vi "Speaker Array Calibration.vi"(11 "folder":path=path "D:/Data/Calibrations/SAL") -> ()   [LabVIEW 2020]
uses:
  SAC Config/SAC Config.xctl
  HRTF VIs/Typedefs/HRTF-Result.ctl
  Typedefs/SAC-Parameters.ctl
  HRTF VIs/Typedefs/HRTF-Waveform.ctl
  HRTF VIs/Typedefs/HRTF-Window.ctl
  HRTF VIs/Typedefs/HRTF-Window Type.ctl
  Typedefs/SAC-State.ctl
  Typedefs/SAC-Options.ctl
  Typedefs/SAC-Hardware Config (TDT).ctl
  PXI DAQ VIs/TDT VIs/Typedefs/TDT-Output source.ctl
  PXI DAQ VIs/TDT VIs/Typedefs/TDT-Device ID.ctl
  PXI DAQ VIs/TDT VIs/Typedefs/TDT-Device Config.ctl
  PXI DAQ VIs/TDT VIs/Typedefs/TDT-Input source.ctl
  HRTF VIs/Typedefs/HRTF-State Machine Action.ctl
  Typedefs/SAC-Runtime Data.ctl
  <vilib>/Analysis/2dsp.llb/Real FFT.vi
  <vilib>/Utility/miscctls.llb/LVBoundsTypeDef.ctl
  <vilib>/Analysis/NI_AALPro.lvlib
panel:
  in  "Measure":bool
  in  "Sensitivity (dB V/SPL)":dbl=128.0
  in  "Mic gain":dbl=128.0
  in  "Compute":bool
  in  "Window":T1={"Window"=0, "Length (ms)"=50.0, "Center (ms)"=50.0} {"Window" items=["None", "Rectangle", "Hanning"]}
  out "Result":T2
  out "StimDur":dbl format="%#_3g ms"
  in  "wftab":enum32{"Page 1", "Page 2"}(tab)
  in  "Freq Step (Hz)":dbl=50.0
  in  "Seed":i32=50
  in  "Order":i32=50
  in  "Attenuation (dB)":dbl=30.0
  in  "Sample Rate (Hz)":dbl=100000.0
  in  "Waveform":enum16{"Chirp", "MLS"}(ring)
  out "Progress":u8(slide) scale=0.0..2.0
  in  "Start":bool
  in  "Stop":bool
  in  "Config":i32(xcontrol)
  in  "Averages":i32=128
  in  "Data Tab":enum32{"Stimulus", "Response", "Calibrations"}(tab)
  out "StimPhase":cluster{i32, "dx":dbl, "Y":dbl[]}(graph)
  out "StimMag":cluster{i32, "dx":dbl, "Y":dbl[]}(graph)
  out "StimAutocorr":cluster{dbl, "dx":dbl, "Y":dbl[]}(graph) caption="Autocorrelation"
  out "Stimulus (time)":cluster{i32, "dx":dbl, "Y":dbl[]}(graph) caption="Amplitude"
  out "RespTime":cluster{"offset":dbl, "dx":dbl, "Y":dbl[]}(graph) caption="Amplitude"
  in  "RespFiles":u16(ring) items=["", "Speaker-az0", "Speaker-az90"]
  out "RespCorr":cluster{"offset":dbl, "dx":dbl, "Y":dbl[]}(graph) caption="Impulse Response"
  out "RespMag":cluster{"offset":dbl, "dx":dbl, "Y":dbl[]}(graph)
  out "RespPhase":cluster{"offset":dbl, "dx":dbl, "Y":dbl[]}(graph)
  out "Status":string
  in  "ASTFFiles":u16(ring) items=["", "Speaker-az-90", "Speaker-az0", "Speaker-az45", "Speaker-az90"]
  out "ASTFMag":cluster{"offset":dbl, "dx":dbl, "Y":dbl[]}(graph)
  out "ASTFPhase":cluster{"offset":dbl, "dx":dbl, "Y":dbl[]}(graph)
  out "ASIR":cluster{"offset":dbl, "dx":dbl, "Y":dbl[]}(graph) caption="Impulse Response"
  # "Speaker Array Calibration"
  # "Stimulus"
  # "ASTF"
  # "Response"
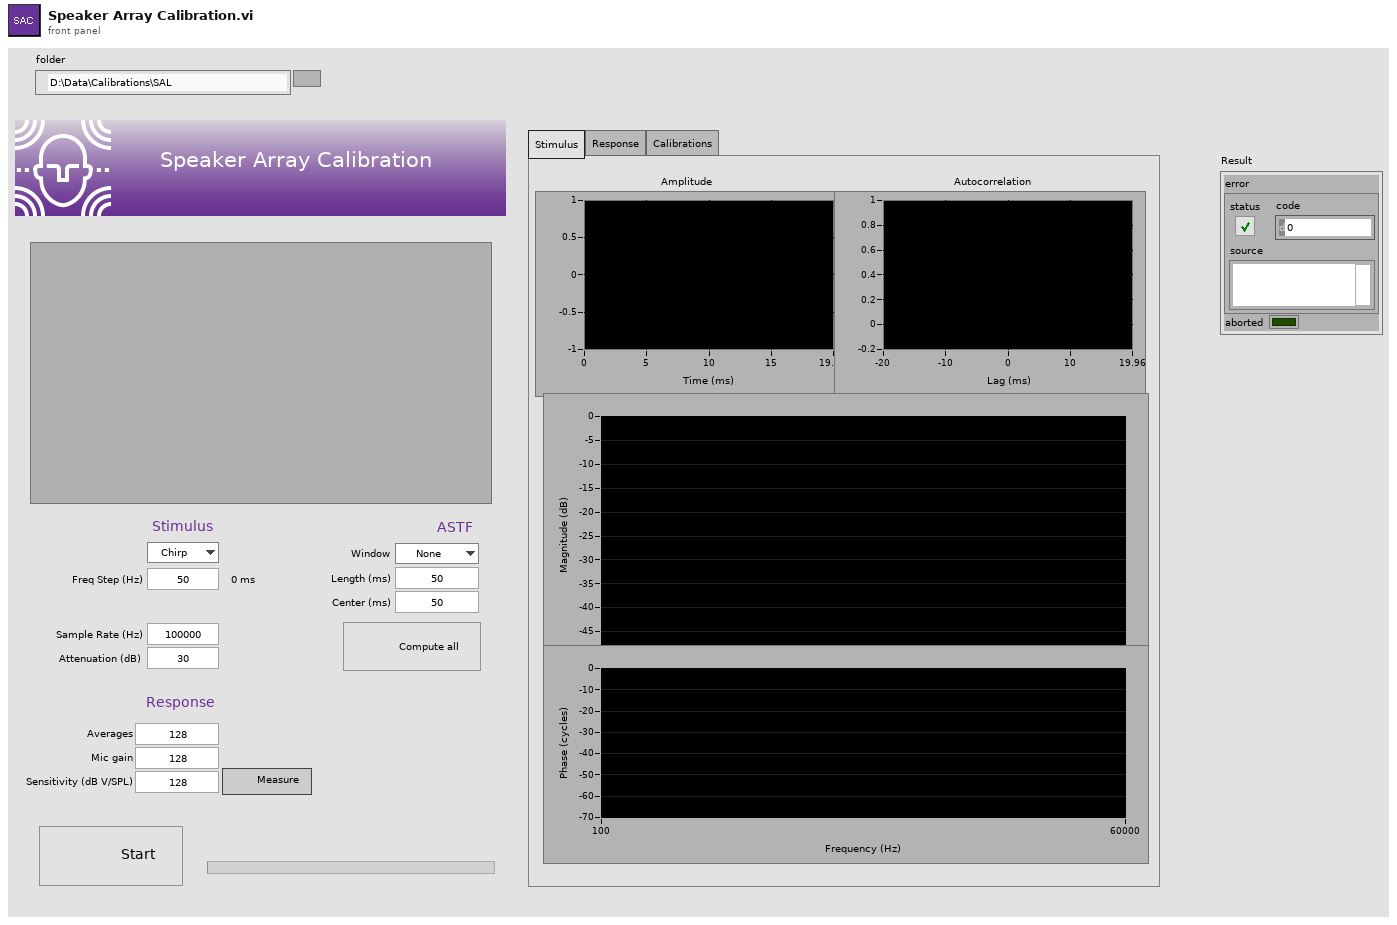
[diagram p1: front panel]
types:
  T1 = cluster{"Window":u16, "Length (ms)":dbl, "Center (ms)":dbl}
  T2 = typedef "HRTF-Result.ctl" = cluster{"error":errorcluster, "aborted":bool}
  T3 = typedef "SAC-Parameters.ctl" = cluster{"Fs (Hz)":dbl, "atten (dB)":dbl, "Waveform":T4, "Freq Res (Hz)":dbl, "Order":i32, "Averages":i32, "seed":i64, "Window":T5, "Mic gain":dbl, "Mic sens":dbl}
  T4 = typedef "HRTF-Waveform.ctl" = enum16{"Chirp", "MLS"}
  T5 = typedef "HRTF-Window.ctl" = cluster{"Type":T6, "Length (ms)":dbl, "Center (ms)":dbl}
  T6 = typedef "HRTF-Window Type.ctl" = enum16{"None", "Rectangle", "Hanning"}
  T7 = typedef "SAC-Options.ctl" = cluster{"Root folder":path, "Wait (s)":dbl, "Azimuths":dbl[]}
  T8 = typedef "SAC-State.ctl" = cluster{"Folder":path, "Elevation":dbl, "iAzimuth":i32, "ID":string, "Azimuth":dbl}
  T9 = typedef "LVBoundsTypeDef.ctl" = cluster{"Width":u32, "Height":u32}
  T10 = enum8{"Enabled", "Disabled", "Disabled and Grayed Out"}
  T11 = typedef "TDT-Device Config.ctl" = cluster{"Output":T12, "Input":T14}
  T12 = typedef "TDT-Output source.ctl" = cluster{"Device":T13, "Num":i32}
  T13 = typedef "TDT-Device ID.ctl" = enum16{"None", "PA5", "RP2", "RL2", "RA16", "RV8", "RX5", "RX6", "RX7", "RX8", "RZ2", "RZ5", "RZ6"}
  T14 = typedef "TDT-Input source.ctl" = enum16{"Front Panel", "RA4LI", "RA16LI"}
  T15 = enum32{"Invalid", "Standard", "Closed", "Hidden", "Minimized", "Maximized"}
  T16 = typedef "SAC-Hardware Config (TDT).ctl" = cluster{"Output":T12, "Speaker":cluster{"Channel":i32, "Primary mux":i32, "Secondary mux":i32}, "Cal mic":i32}
  T17 = typedef "LVRangeTypeDef.ctl" = cluster{"Minimum":dbl, "Maximum":dbl, "Increment":dbl, "Minor Increment":dbl, "Start":dbl}
  T18 = typedef "SAC-Runtime Data.ctl" = cluster{"StimSpec":cdb[], "Mic Sum":dbl[], "df (Hz)":dbl, "dt (ms)":dbl, "Navg":i32, "Nacq":i32, "pts/rep":i32, "reps/frame":i32, "Stimulus":dbl[]}
  T19 = typedef "HRTF-State Machine Action.ctl" = enum16{"Wait", "Init", "Multiplex", "Measure", "Save", "End"}
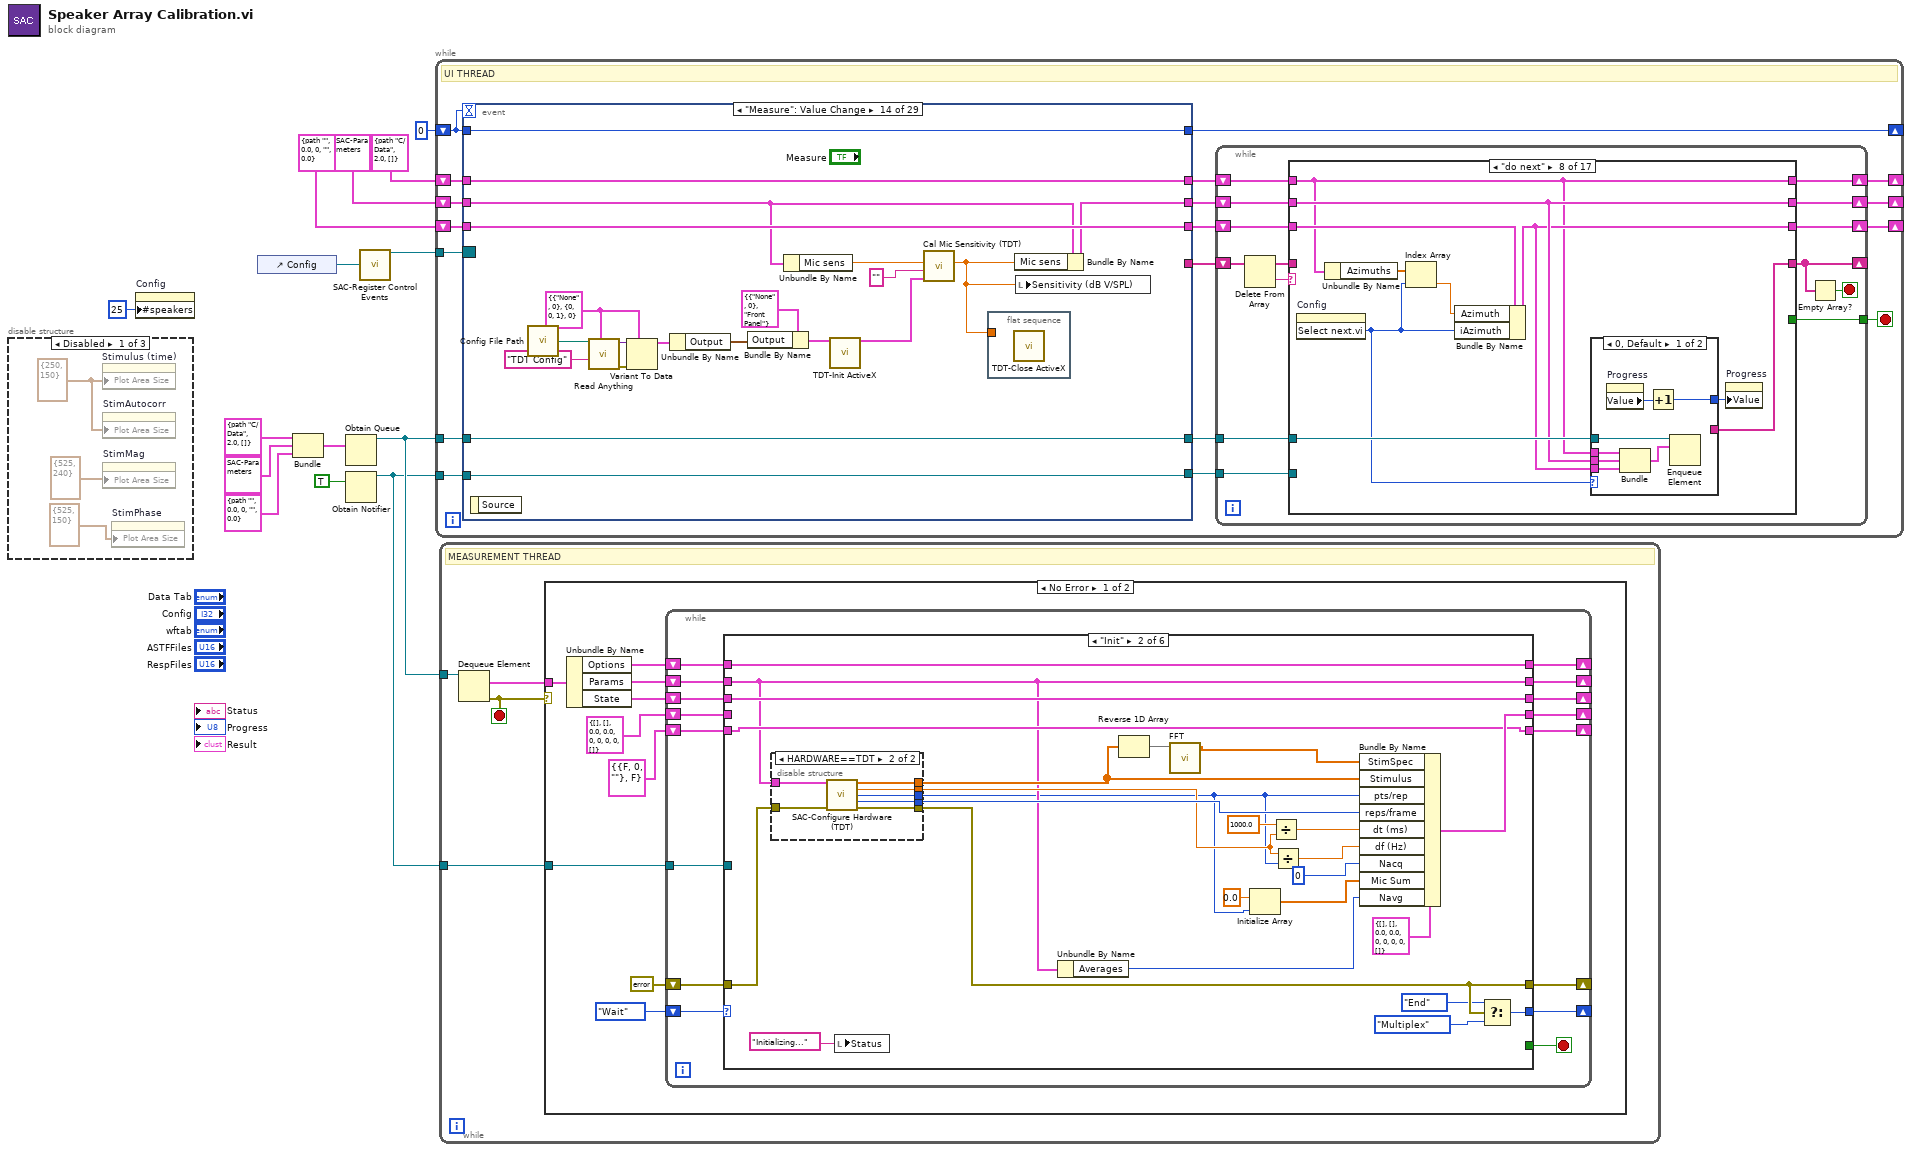
[diagram p0: block diagram]
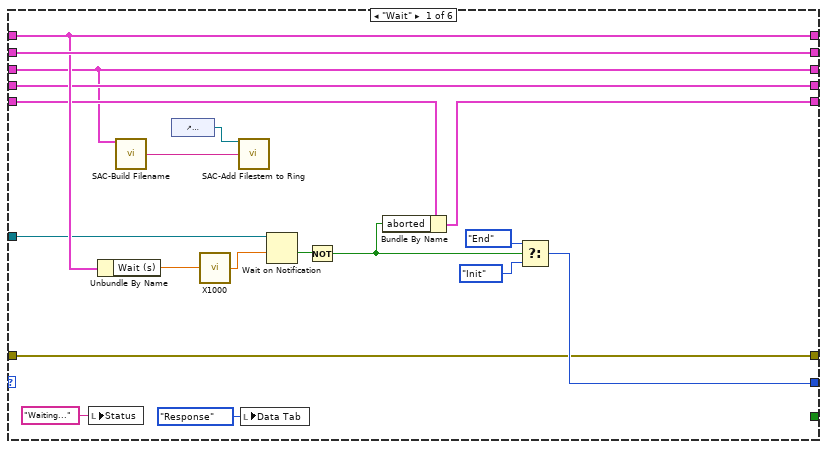
[diagram p2: hidden frame]
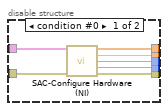
[diagram p3: hidden frame]
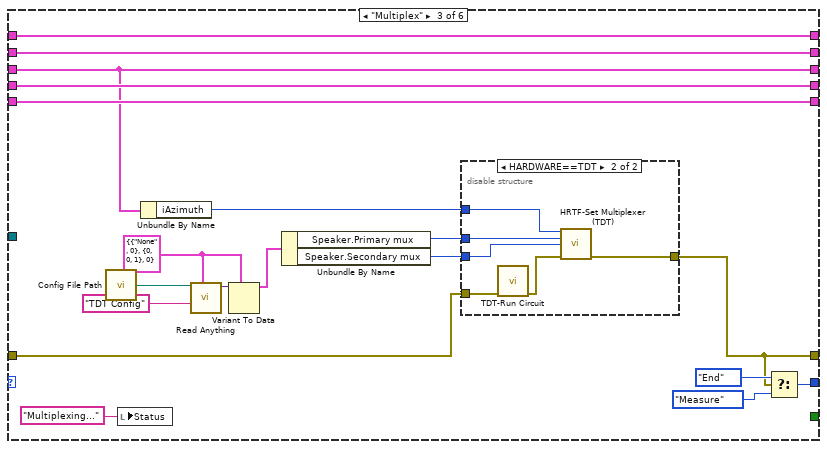
[diagram p4: hidden frame]
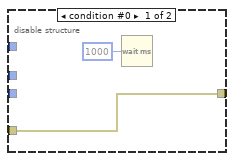
[diagram p5: hidden frame]
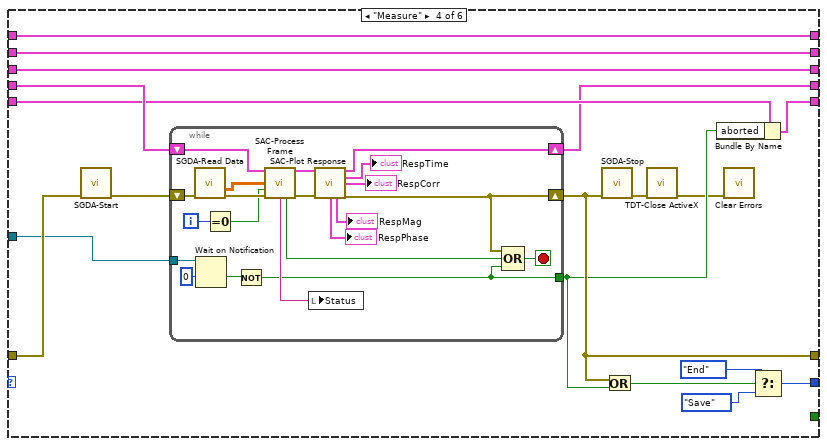
[diagram p6: hidden frame]
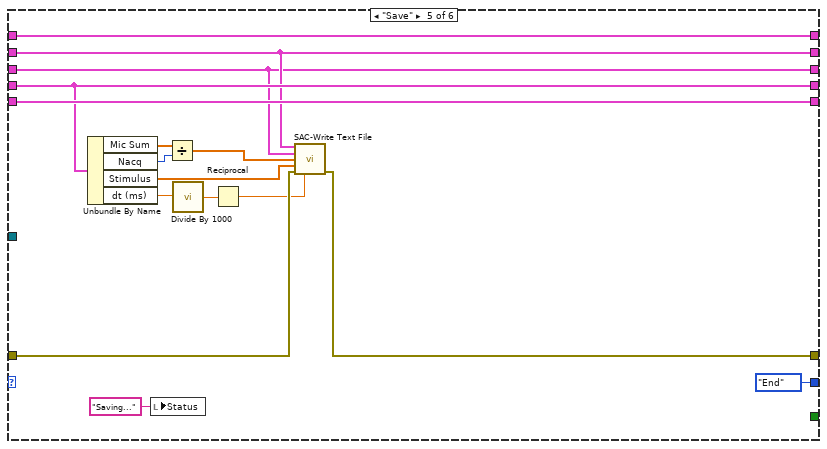
[diagram p7: hidden frame]
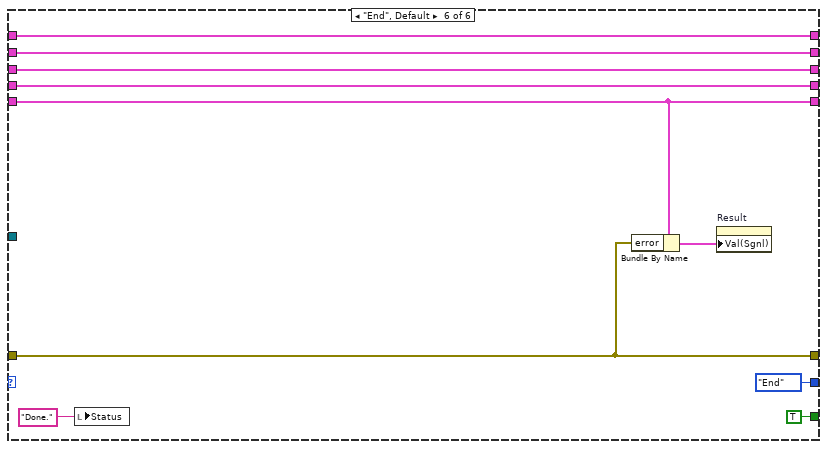
[diagram p8: hidden frame]
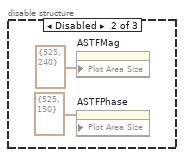
[diagram p10: hidden frame]
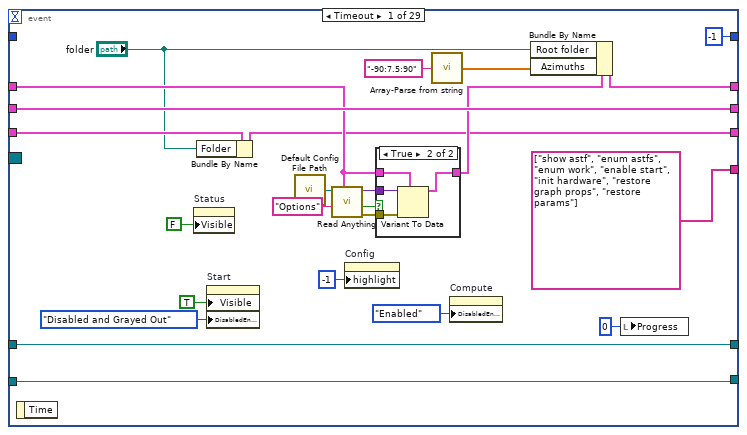
[diagram p12: hidden frame]
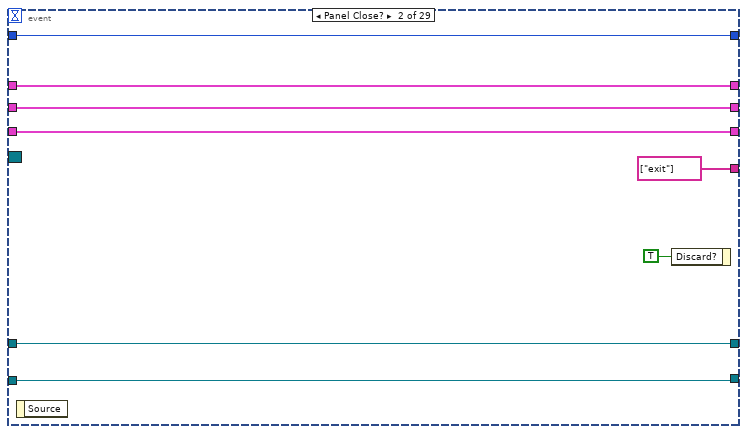
[diagram p14: hidden frame]
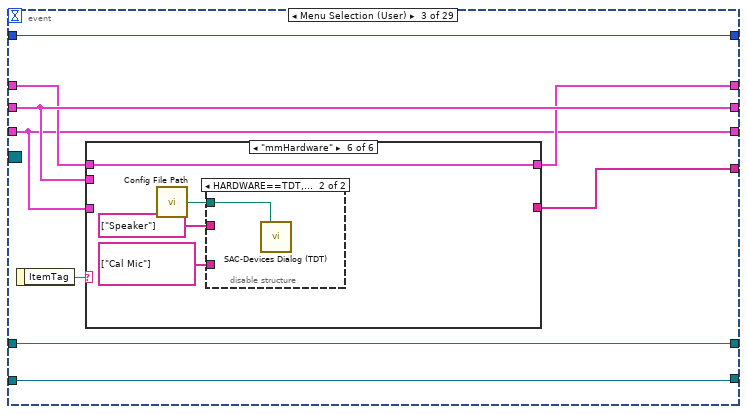
[diagram p15: hidden frame]
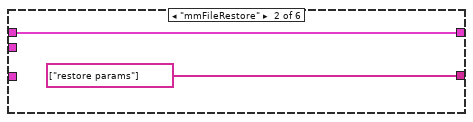
[diagram p17: hidden frame]
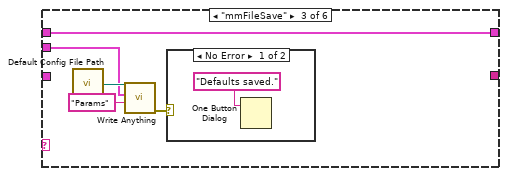
[diagram p18: hidden frame]
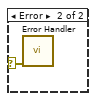
[diagram p19: hidden frame]
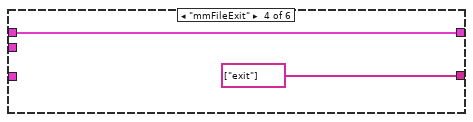
[diagram p20: hidden frame]
diagram:
  n1 = disable-structure shown="Disabled" {
    frame Disabled {
      w17 = T9 {"Width"=250, "Height"=150} ("Plot Area:Size")
      n2 = property on="Stimulus (time)" class="WFGraph (strict)"("Plot Area Size"=w17) -> ()  [unwired: 2 in, 2 out]
      n3 = property on="StimAutocorr" class="WFGraph (strict)"("Plot Area Size"=w17) -> ()  [unwired: 2 in, 2 out]
      n4 = property on="StimMag" class="WFGraph (strict)"("Plot Area Size"=T9 {"Width"=525, "Height"=240} ("Plot Area:Size")) -> ()  [unwired: 2 in, 2 out]
      n5 = property on="StimPhase" class="WFGraph (strict)"("Plot Area Size"=T9 {"Width"=525, "Height"=150} ("Plot Area:Size")) -> ()  [unwired: 2 in, 2 out]
    }
    frame Disabled {
      n6 = property on="ASTFMag" class="WFGraph (strict)"("Plot Area Size"=T9 {"Width"=525, "Height"=240} ("Plot Area:Size")) -> ()  [unwired: 2 in, 2 out]
      n7 = property on="ASTFPhase" class="WFGraph (strict)"("Plot Area Size"=T9 {"Width"=525, "Height"=150} ("Plot Area:Size")) -> ()  [unwired: 2 in, 2 out]
    }
    frame Enabled {
    }
  }
  n8 = property on="Config" class="SAC Config (strict)"("#speakers"=25) -> ()  [unwired: 2 in, 2 out]
  n9 = control-ref of="Config"() -> (w9:refnum<vi>)
  n10 = Bundle("Options"=T7 {"Root folder"=path "C:/Data", "Wait (s)"=2.0, "Azimuths"=[]}, "Params"=T3 {"Fs (Hz)"=100000.0, "atten (dB)"=20.0, "Waveform"=enum."Chirp", "Freq Res (Hz)"=50.0, "Order"=10, "Averages"=100, "seed"=-1, "Window"={"Type"=enum."None", "Length (ms)"=0.0, "Center (ms)"=0.0}, "Mic gain"=0.0, "Mic sens"=0.0}, "State"=T8 {"Folder"=path "", "Elevation"=0.0, "iAzimuth"=0, "ID"="", "Azimuth"=0.0}) -> (w2:cluster{"Options":T7, "Params":T3, "State":T8})  [unwired: 1 in]
  n11 = Obtain Queue(element data type=w2) -> (queue out=w14:refnum<queue>)  [unwired: 4 in, 2 out]
  n12 = Obtain Notifier(notification data type=TRUE) -> (notifier out=w11:refnum<notifier>)  [unwired: 3 in, 2 out]
  n13 = call "SAC-Register Control Events.vi"("Refs"=w9) -> ("Event Registration Refnum"=w1:refnum<event-registration>)  [unwired: 13 in, 1 out]
  n14 = while {
    tunnel: w14 -> [w37]
    shift-right: [w36] -> _
    shift-left: 0 -> [w35]
    shift-right: [w26] -> _
    shift-left: T3 {"Fs (Hz)"=100000.0, "atten (dB)"=20.0, "Waveform"=enum."Chirp", "Freq Res (Hz)"=50.0, "Order"=10, "Averages"=100, "seed"=-1, "Window"={"Type"=enum."None", "Length (ms)"=5.0, "Center (ms)"=2.5}, "Mic gain"=0.0, "Mic sens"=0.0} ("Params") -> [w34]
    tunnel: w11 -> [w33]
    shift-right: [w25] -> _
    shift-left: T7 {"Root folder"=path "C:/Data", "Wait (s)"=2.0, "Azimuths"=[]} ("Options") -> [w32]
    shift-right: [w27] -> _
    shift-left: T8 {"Folder"=path "", "Elevation"=0.0, "iAzimuth"=0, "ID"="", "Azimuth"=0.0} ("State") -> [w31]
    tunnel: w1 -> [w21]
    stop <- w24 stop-if-true
    # "UI THREAD"
    n15 = event shown="[13] \"Measure\": Value Change" {
      selector: w21 -> [_ _ _ _ _ _ _ _ _ _ _ _ _ _ _ _ _ _ _ _ _ _ _ _ _ _ _ _ _]
      dyn-events: _ -> [_ _ _ _ _ _ _ _ _ _ _ _ _ _ _ _ _ _ _ _ _ _ _ _ _ _ _ _ _]
      timeout: w35 -> [_ _ _ _ _ _ _ _ _ _ _ _ _ _ _ _ _ _ _ _ _ _ _ _ _ _ _ _ _]
      tunnel: w37 -> [w55 w68 w79 w115 w123 w132 w141 w150 w159 w167 w174 w183 w191 w213 w221 w229 w237 w255 w256 w266 w285 w296 w307 w315 w322 w335 w355 w370 w378]
      tunnel: [-1 w74 w82 w118 w128 w137 w146 w155 w164 w172 w180 w188 w196 w216 w225 w233 w241 w254 w262 w271 w289 w300 w311 w319 w326 w339 w359 w374 w382] -> w36
      tunnel: w35 -> [_ w74 w82 w118 w128 w137 w146 w155 w164 w172 w180 w188 w196 w216 w225 w233 w241 w254 w262 w271 w289 w300 w311 w319 w326 w339 w359 w374 w382]
      tunnel: w34 -> [w57 w73 w81 w117 w125 w134 w143 w152 w161 w169 w176 w185 w193 w211 w224 w232 w240 w253 w261 w270 w288 w299 w310 w318 w325 w338 w358 w373 w381]
      tunnel: [w57 w73 w81 w117 w124 w133 w142 w151 w160 w168 w175 w184 w192 w210 w219 w227 w235 w253 w261 w270 w288 w299 w310 w318 w325 w338 w358 w373 w381] -> w29
      tunnel: w33 -> [w54 w67 w78 w114 w122 w131 w140 w149 w158 w166 w173 w182 w190 w212 w220 w228 w236 w252 w260 w265 w284 w295 w306 w314 w321 w334 w354 w369 w377]
      tunnel: w32 -> [w49 w70 w77 w116 w127 w136 w145 w154 w163 w171 w178 w187 w195 w215 w223 w231 w239 w250 w257 w267 w287 w298 w309 w317 w324 w337 w357 w372 w380]
      tunnel: w31 -> [w56 w71 w75 w113 w126 w135 w144 w153 w162 w170 w177 w186 w194 w214 w222 w230 w238 w251 w258 w268 w286 w297 w308 w316 w323 w336 w356 w371 w379]
      tunnel: [w40 w70 w76 w116 w127 w136 w145 w154 w163 w171 w178 w187 w195 w215 w223 w231 w239 w250 w257 w267 w287 w298 w309 w317 w324 w337 w357 w372 w380] -> w20
      tunnel: [w39 w71 w75 w113 w126 w135 w144 w153 w162 w170 w177 w186 w194 w214 w222 w230 w238 w251 w258 w268 w286 w297 w308 w316 w323 w336 w356 w371 w379] -> w28
      tunnel: [string[] ["show astf", "enum astfs", "enum work", "enable start", "init hardware", "restore graph props", "restore params"] string[] ["exit"] w80 string[] ["enable start"] ("String") string[] ["plot stim"] ("String") string[] ["plot stim"] ("String") string[] ["plot stim"] ("String") string[] ["plot stim"] ("String") string[] ["plot stim"] ("String") _ _ _ _ _ string[] ["update window"] ("String") _ _ string[] ["do next"] ("String") _ w264 _ _ _ string[] ["read work"] ("String") string[] ["read astf"] ("String") w328 w348 _ string[] ["compute"] ("String")] -> w30
      tunnel: [w55 w68 w79 w115 w123 w132 w141 w150 w159 w167 w174 w183 w191 w213 w221 w229 w237 w255 w256 w266 w285 w296 w307 w315 w322 w335 w355 w370 w378] -> w23
      tunnel: [w54 w67 w78 w114 w122 w131 w140 w149 w158 w166 w173 w182 w190 w212 w220 w228 w236 w248 w260 w265 w284 w295 w306 w314 w321 w334 w354 w369 w377] -> w22
      event Timeout {
        n16 = event-data() -> ()  [unwired: 1 in, 1 out]
        n17 = property on="Status" class="Str"("Visible"=FALSE) -> ()  [unwired: 2 in, 2 out]
        n18 = Bundle By Name(cluster=w56, "Folder"="folder") -> (w39:T8)
        n19 = property on="Start" class="Bool"("Visible"=TRUE, "DisabledEnum"=T10."Disabled and Grayed Out" ("Disabled")) -> ()  [unwired: 2 in, 2 out]
        n20 = call "Default Config File Path.vi"() -> ("Default config file name"=w52:path)
        n21 = call "Read Anything.vi"("Type of Anything"=w49, "Section Name (Name of \"Type of Anything\")"="Options" ("Section Name (Name of \"Type of Anything\")"), "Path (dialog)"=w52) -> ("Error Out"=w53:errorcluster, "Found?"=w51:bool, "Anything"=w50:variant)  [unwired: 6 in]
        n22 = property on="Config" class="SAC Config (strict)"("highlight"=-1) -> ()  [unwired: 2 in, 2 out]
        n23 = case shown="True" w51 {
          tunnel: w53 -> [_ w66]
          tunnel: w50 -> [_ w65]
          tunnel: w49 -> [w62 w64]
          tunnel: [w62 w63] -> w48
          frame False {
          }
          frame True {
            n24 = Variant To Data(error in=w66, type=w64, Variant=w65) -> (data=w63:T7)  [unwired: 1 out]
          }
        }
        n25 = call "Array-Parse from string.vi"("String"="-90:7.5:90") -> ("Array"=w43:dbl[])  [unwired: 13 in, 1 out]
        n26 = property on="Compute" class="Bool"("DisabledEnum"=T10."Enabled" ("Disabled")) -> ()  [unwired: 2 in, 2 out]
        n27 = Bundle By Name(cluster=w48, "Root folder"="folder", "Azimuths"=w43) -> (w40:T7)
        n28 = local write "Progress"(u8 0 ("Progress")) -> ()
      }
      event Panel Close? {
        n29 = event-data() -> ()  [unwired: 1 in, 1 out]
        n30 = event-data("Discard?"=TRUE) -> ()  [unwired: 1 in, 1 out]
      }
      event Menu Selection (User) {
        n31 = event-data() -> ("ItemTag"=w83:string)  [unwired: 1 in]
        n32 = case shown="\"mmHardware\"" w83 {
          tunnel: w81 -> [_ _ w89 _ _ _]
          tunnel: [_ string[] ["restore params"] _ string[] ["exit"] w96 _] -> w80
          tunnel: w77 -> [w84 w85 w87 w94 w99 w107]
          tunnel: [w84 w85 w87 w94 w97 w107] -> w76
          tunnel: w75 -> [_ _ _ _ _ _]
          frame "False", Default {
          }
          frame "mmFileRestore" {
          }
          frame "mmFileSave" {
            n33 = call "Default Config File Path.vi"() -> ("Default config file name"=w91:path)
            n34 = call "Write Anything.vi"("Section Name (Name of \"Anything\")"="Params" ("Section Name (Name of \"Anything\")"), "Anything"=w89, "Path (dialog)"=w91) -> ("Error Out"=w88:errorcluster)  [unwired: 7 in, 1 out]
            n35 = case shown="No Error" w88 {
              selector: w88 -> [_ w93]
              frame No Error {
                n36 = One Button Dialog(message="Defaults saved.") -> ()  [unwired: 1 in, 1 out]
              }
              frame Error {
                n37 = call "Error Handler.vi"("error in (no error)"=w93) -> ()  [unwired: 13 in, 2 out]
              }
            }
          }
          frame "mmFileExit" {
          }
          frame "mmOptions" {
            n38 = call "SAC-Options Dialog.vi"("Options in"=w99) -> ("Options out"=w97:T7, "Canceled?"=w98:bool)  [unwired: 13 in]
            n39 = case shown="False" w98 {
              tunnel: w97 -> [w101 _]
              tunnel: [string[] ["apply options"] ("String") _] -> w96
              frame False {
                n40 = call "Default Config File Path.vi"() -> ("Default config file name"=w103:path)
                n41 = call "Write Anything.vi"("Section Name (Name of \"Anything\")"="Options" ("Section Name (Name of \"Anything\")"), "Anything"=w101, "Path (dialog)"=w103) -> ()  [unwired: 7 in, 2 out]
              }
              frame True {
              }
            }
          }
          frame "mmHardware" {
            n42 = call "Config File Path.vi"() -> ("Default config file name"=w104:path)  [unwired: 1 in]
            n43 = disable-structure shown="HARDWARE==TDT, Default" {
              disable-tunnel: string[] ["Speaker"] ("Custom Outputs") -> [w110 _]
              disable-tunnel: string[] ["Cal Mic"] ("Custom Outputs") -> [w109 _]
              disable-tunnel: w104 -> [w108 w111]
              frame condition #0 {
                n44 = call "Connection Manager (general).vi"("Path"=w108, "Custom Inputs"=w109, "Custom Outputs"=w110) -> ()  [unwired: 8 in, 1 out]
              }
              frame condition #1 (active) {
                n45 = call "SAC-Devices Dialog (TDT).vi"("Path"=w111) -> ()  [unwired: 14 in, 1 out]
              }
            }
          }
        }
      }
      event User Event {
        n46 = event-data() -> ()  [unwired: 1 in, 1 out]
      }
      event "Waveform": Value Change {
        n47 = event-data() -> ()  [unwired: 1 in, 1 out]
        n48 = Bundle By Name(cluster=w125, "Waveform"="Waveform") -> (w124:T3)
        n49 = To Long Integer(number="Waveform") -> (32bit integer=w120:i32)
        n50 = local write "wftab"(w120) -> ()
      }
      event "Freq Step (Hz)": Value Change {
        n51 = event-data() -> ()  [unwired: 1 in, 1 out]
        n52 = Bundle By Name(cluster=w134, "Freq Res (Hz)"="Freq Step (Hz)") -> (w133:T3)
      }
      event "Order": Value Change {
        n53 = event-data() -> ()  [unwired: 1 in, 1 out]
        n54 = Bundle By Name(cluster=w143, "Order"="Order") -> (w142:T3)
      }
      event "Seed": Value Change {
        n55 = event-data() -> ()  [unwired: 1 in, 1 out]
        n56 = Bundle By Name(cluster=w152, "seed"="Seed") -> (w151:T3)
      }
      event "Sample Rate (Hz)": Value Change {
        n57 = event-data() -> ()  [unwired: 1 in, 1 out]
        n58 = Bundle By Name(cluster=w161, "Fs (Hz)"="Sample Rate (Hz)") -> (w160:T3)
      }
      event "Attenuation (dB)": Value Change {
        n59 = event-data() -> ()  [unwired: 1 in, 1 out]
        n60 = Bundle By Name(cluster=w169, "atten (dB)"="Attenuation (dB)") -> (w168:T3)
      }
      event "Averages": Value Change {
        n61 = event-data() -> ()  [unwired: 1 in, 1 out]
        n62 = Bundle By Name(cluster=w176, "Averages"="Averages") -> (w175:T3)
      }
      event "Mic gain": Value Change {
        n63 = event-data() -> ()  [unwired: 1 in, 1 out]
        n64 = Bundle By Name(cluster=w185, "Mic gain"="Mic gain") -> (w184:T3)
      }
      event "Sensitivity (dB V/SPL)": Value Change {
        n65 = event-data() -> ()  [unwired: 1 in, 1 out]
        n66 = Bundle By Name(cluster=w193, "Mic sens"="Sensitivity (dB V/SPL)") -> (w192:T3)
      }
      event "Measure": Value Change {
        w205 = T16 {"Output"={"Device"=enum."None", "Num"=0}, "Speaker"={"Channel"=0, "Primary mux"=0, "Secondary mux"=1}, "Cal mic"=0} ("TDT")
        n67 = event-data() -> ()  [unwired: 1 in, 1 out]
        n68 = call "Config File Path.vi"() -> ("Default config file name"=w204:path)  [unwired: 1 in]
        n69 = call "Read Anything.vi"("Type of Anything"=w205, "Section Name (Name of \"Type of Anything\")"="TDT Config" ("Section Name (Name of \"Type of Anything\")"), "Path (dialog)"=w204) -> ("Error Out"=w201:errorcluster, "Anything"=w202:variant)  [unwired: 6 in, 1 out]
        n70 = Variant To Data(error in=w201, type=w205, Variant=w202) -> (data=w198:T16)  [unwired: 1 out]
        n71 = Unbundle By Name(w198) -> ("Output"=w199:T12)
        n72 = Bundle By Name(cluster=T11 {"Output"={"Device"=enum."None", "Num"=0}, "Input"=enum."Front Panel"} ("TDT-Device Config"), "Output"=w199) -> (w197:T11)
        n73 = Unbundle By Name(w211) -> ("Mic sens"=w209:dbl)
        n74 = call "TDT-Init ActiveX.vi"("TDT-Device Config"=w197) -> ("TDT-Device Config out"=w207:T11)  [unwired: 11 in, 3 out]
        n75 = call "Cal Mic Sensitivity (TDT).vi"("Device Config"=w207, "User ID"="", "Mic Sens (dB V/SPL) in"=w209) -> ("Mic Sens (dB V/SPL)"=w206:dbl)  [unwired: 8 in]
        n76 = flat-sequence {
          tunnel: w206 -> [_]
          frame #0 {
            n77 = call "TDT-Close ActiveX.vi"() -> ()  [unwired: 15 in, 1 out]
          }
        }
        n78 = Bundle By Name(cluster=w211, "Mic sens"=w206) -> (w210:T3)
        n79 = local write "Sensitivity (dB V/SPL)"(w206) -> ()
      }
      event "Window.Window": Value Change {
        n80 = event-data() -> ("NewVal"=w217:u16)  [unwired: 1 in]
        n81 = Bundle By Name(cluster=w224, "Window.Type"=w217) -> (w219:T3)
      }
      event "Window.Length (ms)": Value Change {
        n82 = event-data() -> ("NewVal"=w226:dbl)  [unwired: 1 in]
        n83 = Bundle By Name(cluster=w232, "Window.Length (ms)"=w226) -> (w227:T3)
      }
      event "Window.Center (ms)": Value Change {
        n84 = event-data() -> ("NewVal"=w234:dbl)  [unwired: 1 in]
        n85 = Bundle By Name(cluster=w240, "Window.Center (ms)"=w234) -> (w235:T3)
      }
      event "Start": Value Change {
        n86 = event-data() -> ()  [unwired: 1 in, 1 out]
        n87 = Cancel Notification(0:w252) -> (8:w248:refnum<notifier>)  [unwired: 1 in, 2 out]
        n88 = property on="Config" class="SAC Config (strict)"() -> ("selection"=w247:i32[])  [unwired: 2 in, 2 out]
        n89 = Array Size(array=w247) -> (size(s)=w246:i32)
        n90 = property on="Progress" class="Slide (strict)"("Scale.Maximum"=w246, "Value"=u8 0 ("Progress")) -> ()  [unwired: 2 in, 2 out]
        n91 = property on="RespFiles" class="Ring (strict)"("DisabledEnum"=T10."Disabled and Grayed Out" ("Disabled")) -> ()  [unwired: 2 in, 2 out]
        n92 = property on="Status" class="Str"("Visible"=TRUE) -> ()  [unwired: 2 in, 2 out]
        n93 = property on="Start" class="Bool"("Visible"=FALSE) -> ()  [unwired: 2 in, 2 out]
      }
      event "Stop": Value Change {
        n94 = event-data() -> ()  [unwired: 1 in, 1 out]
        n95 = Send Notification(notification=TRUE ("element"), notifier=w260) -> ()  [unwired: 1 in, 2 out]
      }
      event Value Change {
        n96 = event-data() -> ("NewVal.error"=w269:errorcluster, "NewVal.aborted"=w263:bool)  [unwired: 1 in]
        n97 = case shown="No Error" w269 {
          selector: w269 -> [_ w279]
          tunnel: [w273 string[] ["end run"] ("String")] -> w264
          tunnel: w263 -> [w272 _]
          frame No Error {
            n98 = case shown="False" w272 {
              tunnel: [w275 string[] ["end run"] ("String")] -> w273
              frame False {
                n99 = Build Array("do next", "update" ("String")) -> (w275:string[])
              }
              frame True {
              }
            }
          }
          frame Error {
            n100 = call "Error Handler.vi"("error in (no error)"=w279) -> ()  [unwired: 13 in, 2 out]
          }
        }
      }
      event "StimPhase": Scale Range Change {
        n101 = event-data() -> ("ScaleRef"=w283:refnum<vi>, "NewRange"=w280:T17)  [unwired: 1 in]
        n102 = property on="StimPhase" class="WFGraph (strict)"() -> ("XScale"=w282:refnum<vi>)  [unwired: 2 in, 2 out]
        n103 = Equal?(x=w282, y=w283) -> (x = y?=w281:bool)
        n104 = case shown="True" w281 {
          tunnel: w280 -> [_ w290]
          frame False {
          }
          frame True {
            n105 = property on="StimMag" class="WFGraph (strict)"("XScale.Range"=w290) -> ()  [unwired: 2 in, 2 out]
          }
        }
      }
      event "RespPhase": Scale Range Change {
        n106 = event-data() -> ("ScaleRef"=w294:refnum<vi>, "NewRange"=w291:T17)  [unwired: 1 in]
        n107 = property on="RespPhase" class="WFGraph (strict)"() -> ("XScale"=w293:refnum<vi>)  [unwired: 2 in, 2 out]
        n108 = Equal?(x=w293, y=w294) -> (x = y?=w292:bool)
        n109 = case shown="True" w292 {
          tunnel: w291 -> [_ w301]
          frame False {
          }
          frame True {
            n110 = property on="RespMag" class="WFGraph (strict)"("XScale.Range"=w301) -> ()  [unwired: 2 in, 2 out]
          }
        }
      }
      event "ASTFPhase": Scale Range Change {
        n111 = event-data() -> ("ScaleRef"=w305:refnum<vi>, "NewRange"=w302:T17)  [unwired: 1 in]
        n112 = property on="ASTFPhase" class="WFGraph (strict)"() -> ("XScale"=w304:refnum<vi>)  [unwired: 2 in, 2 out]
        n113 = Equal?(x=w304, y=w305) -> (x = y?=w303:bool)
        n114 = case shown="True" w303 {
          tunnel: w302 -> [_ w312]
          frame False {
          }
          frame True {
            n115 = property on="ASTFMag" class="WFGraph (strict)"("XScale.Range"=w312) -> ()  [unwired: 2 in, 2 out]
          }
        }
      }
      event "RespFiles": Value Change {
        n116 = event-data() -> ()  [unwired: 1 in, 1 out]
      }
      event "ASTFFiles": Value Change {
        n117 = event-data() -> ()  [unwired: 1 in, 1 out]
      }
      event "ASTFFiles": Mouse Wheel {
        n118 = event-data() -> ("Delta"=w330:i32)  [unwired: 1 in]
        n119 = property on="ASTFFiles" class="Ring (strict)"() -> ("Value"=w331:u16, "Strings []"=w332:string[])  [unwired: 2 in, 2 out]
        n120 = Array Size(array=w332) -> (size(s)=w329:i32)
        n121 = Decrement(x=w329) -> (x-1=w327:i32)
        n122 = Greater Than 0?(x=w327) -> (x > 0?=w333:bool)
        n123 = case shown="True" w333 {
          tunnel: w331 -> [_ w346]
          tunnel: w330 -> [_ w345]
          tunnel: w327 -> [_ w343]
          tunnel: [_ string[] ["read astf"] ("String")] -> w328
          frame False {
          }
          frame True {
            n124 = Subtract(x=w346, y=w345) -> (x-y=w344:i32)
            n125 = In Range and Coerce(upper limit=w343, x=w344, lower limit=1) -> (coerced(x)=w341:i32)  [unwired: 1 out]
            n126 = local write "ASTFFiles"(w341) -> ()
          }
        }
      }
      event "RespFiles": Mouse Wheel {
        n127 = event-data() -> ("Delta"=w350:i32)  [unwired: 1 in]
        n128 = property on="RespFiles" class="Ring (strict)"() -> ("Value"=w351:u16, "Strings []"=w352:string[])  [unwired: 2 in, 2 out]
        n129 = Array Size(array=w352) -> (size(s)=w349:i32)
        n130 = Decrement(x=w349) -> (x-1=w347:i32)
        n131 = Greater Than 0?(x=w347) -> (x > 0?=w353:bool)
        n132 = case shown="True" w353 {
          tunnel: w351 -> [_ w366]
          tunnel: w350 -> [_ w365]
          tunnel: w347 -> [_ w363]
          tunnel: [_ string[] ["read work"] ("String")] -> w348
          frame False {
          }
          frame True {
            n133 = Subtract(x=w366, y=w365) -> (x-y=w364:i32)
            n134 = In Range and Coerce(upper limit=w363, x=w364, lower limit=1) -> (coerced(x)=w361:i32)  [unwired: 1 out]
            n135 = local write "RespFiles"(w361) -> ()
          }
        }
      }
      event "ASTFMag": Scale Range Change {
        n136 = event-data() -> ("CtlRef"=w368:refnum<vi>)  [unwired: 1 in]
        n137 = call "Config File Path.vi"() -> ("Default config file name"=w367:path)  [unwired: 1 in]
        n138 = call "Write Graph Properties.vi"("Config File"=w367, "WFGraph Refnum"=w368) -> ()  [unwired: 13 in, 1 out]
      }
      event "Compute": Value Change {
        w375 = T10."Disabled and Grayed Out" ("Disabled")
        n139 = event-data() -> ()  [unwired: 1 in, 1 out]
        n140 = property on="Compute" class="Bool"("DisabledEnum"=w375) -> ()  [unwired: 2 in, 2 out]
        n141 = property on="Start" class="Bool"("DisabledEnum"=w375) -> ()  [unwired: 2 in, 2 out]
      }
    }
    n142 = while {
      shift-right: [w387] -> _
      shift-left: w30 -> [w396]
      shift-right: [w390] -> w25
      shift-left: w20 -> [w393]
      shift-right: [w389] -> w26
      shift-left: w29 -> [w392]
      shift-right: [w388] -> w27
      shift-left: w28 -> [w391]
      tunnel: [w385] -> w24
      tunnel: w23 -> [w384]
      tunnel: w22 -> [w383]
      stop <- w386 stop-if-true
      n143 = Delete From Array(array=w396) -> (deleted portion=w395:string, array with subset deleted=w394:string[])  [unwired: 2 in]
      n144 = case shown="\"do next\"" w395 {
        tunnel: w394 -> [w397 _ w409 w428 w453 w465 w475 _ w502 w513 w523 w533 w547 w567 w578 w590 w603]
        tunnel: w393 -> [w400 w407 w412 w431 w455 w467 w477 w481 w499 w512 w522 w535 w549 w569 w581 w592 w604]
        tunnel: w392 -> [w399 w406 w411 w430 w448 w464 w474 w486 w503 w514 w524 w534 w548 w568 w580 w591 w601]
        tunnel: w391 -> [w398 w405 w410 w429 w454 w466 w476 w485 w500 w505 w515 w529 w546 w566 w579 w584 w593]
        tunnel: [w400 w407 w412 w431 w455 w467 w477 w481 w499 w512 w522 w535 w549 w569 w581 w592 w604] -> w390
        tunnel: [w399 w406 w411 w430 w447 w464 w474 w486 w503 w514 w524 w534 w548 w568 w580 w591 w601] -> w389
        tunnel: [w398 w405 w410 w429 w454 w466 w476 w484 w500 w505 w515 w529 w546 w566 w579 w584 w593] -> w388
        tunnel: [w397 string[] [] w409 w428 w439 w465 w475 w483 w502 w513 w523 w533 w547 w562 w578 w590 w596] -> w387
        tunnel: [_ TRUE _ _ _ _ _ _ _ _ _ _ _ _ _ _ _] -> w385
        tunnel: w384 -> [_ w402 _ _ _ _ _ w487 _ _ _ _ _ _ _ _ _]
        tunnel: w383 -> [_ w401 _ _ _ _ _ _ _ _ _ _ _ _ _ _ _]
        frame "", Default {
        }
        frame "exit" {
          n145 = Release Queue(queue=w402) -> ()  [unwired: 2 in, 3 out]
          n146 = Release Notifier(notifier=w401) -> ()  [unwired: 2 in, 3 out]
          n147 = disable-structure shown="Disabled" {
            frame Disabled {
              n148 = disable-structure shown="HARDWARE==TDT" {
                disable-tunnel: [_ w408] -> _
                frame condition #0 {
                  n149 = call "Abort notifier.vi"() -> ()  [unwired: 6 in, 2 out]
                }
                frame condition #1 (active) {
                  n150 = call "TDT-Close ActiveX.vi"() -> ("error out"=w408:errorcluster)  [unwired: 15 in]
                }
              }
            }
            frame Enabled {
            }
          }
        }
        frame "init hardware" {
          n151 = disable-structure shown="Disabled" {
            frame Disabled {
              n152 = disable-structure shown="HARDWARE==TDT" {
                frame condition #0 {
                  n153 = vi-ref "PXI DAQ Server.vi"() -> (w414:refnum<vi>)
                  n154 = call "Spawn VI.vi"("State"=T15."Hidden", "VI reference"=w414) -> ()  [unwired: 8 in, 2 out]
                }
                frame condition #1 (active) {
                  w418 = T16 {"Output"={"Device"=enum."None", "Num"=0}, "Speaker"={"Channel"=0, "Primary mux"=0, "Secondary mux"=1}, "Cal mic"=0} ("TDT")
                  n155 = call "Config File Path.vi"() -> ("Default config file name"=w419:path)  [unwired: 1 in]
                  n156 = call "Read Anything.vi"("Type of Anything"=w418, "Section Name (Name of \"Type of Anything\")"="TDT Config" ("Section Name (Name of \"Type of Anything\")"), "Path (dialog)"=w419) -> ("Error Out"=w422:errorcluster, "Anything"=w421:variant)  [unwired: 6 in, 1 out]
                  n157 = Variant To Data(error in=w422, type=w418, Variant=w421) -> (data=w423:T16, error out=w424:errorcluster)
                  n158 = Unbundle By Name(w423) -> ("Output"=w415:T12)
                  n159 = Bundle By Name(cluster=T11 {"Output"={"Device"=enum."None", "Num"=0}, "Input"=enum."Front Panel"} ("TDT-Device Config"), "Output"=w415) -> (w416:T11)
                  n160 = call "TDT-Init ActiveX.vi"("TDT-Device Config"=w416, "error in (no error)"=w424) -> ("error out"=w425:errorcluster)  [unwired: 10 in, 3 out]
                  n161 = call "Error Handler.vi"("error in (no error)"=w425) -> ()  [unwired: 13 in, 2 out]
                }
              }
            }
            frame Enabled {
            }
          }
        }
        frame "restore graph props" {
          n162 = control-ref of="ASTFMag"() -> (w426:refnum<vi>)
          n163 = call "Default Config File Path.vi"() -> ("Default config file name"=w427:path)
          n164 = call "Read Graph Properties.vi"("Config File"=w427, "WFGraph Refnum"=w426) -> ()  [unwired: 12 in, 2 out]
        }
        frame "restore params" {
          n165 = call "Default Config File Path.vi"() -> ("Default config file name"=w451:path)
          n166 = call "Read Anything.vi"("Type of Anything"=w448, "Section Name (Name of \"Type of Anything\")"="Params" ("Section Name (Name of \"Type of Anything\")"), "Path (dialog)"=w451) -> ("Error Out"=w452:errorcluster, "Found?"=w450:bool, "Anything"=w449:variant)  [unwired: 6 in]
          n167 = case shown="True" w450 {
            tunnel: w452 -> [_ w460]
            tunnel: w449 -> [_ w459]
            tunnel: w448 -> [w456 w458]
            tunnel: [w456 w457] -> w447
            frame False {
            }
            frame True {
              n168 = Variant To Data(error in=w460, type=w458, Variant=w459) -> (data=w457:T3)  [unwired: 1 out]
            }
          }
          n169 = Unbundle By Name(w447) -> ("Fs (Hz)"=w446:dbl, "atten (dB)"=w445:dbl, "Waveform"=w440:T4, "Freq Res (Hz)"=w444:dbl, "Order"=w441:i32, "Averages"=w443:i32, "seed"=w436:i64, "Window"=w435:T5, "Mic gain"=w433:dbl, "Mic sens"=w432:dbl)
          n170 = local write "Sensitivity (dB V/SPL)"(w432) -> ()
          n171 = local write "Mic gain"(w433) -> ()
          n172 = local write "Window"(w435) -> ()
          n173 = local write "Sample Rate (Hz)"(w446) -> ()
          n174 = local write "Attenuation (dB)"(w445) -> ()
          n175 = local write "Waveform"(w440) -> ()
          n176 = local write "Freq Step (Hz)"(w444) -> ()
          n177 = local write "Averages"(w443) -> ()
          n178 = local write "Seed"(w436) -> ()
          n179 = local write "Order"(w441) -> ()
          n180 = To Long Integer(number=w440) -> (32bit integer=w437:i32)
          n181 = Build Array (concatenate)("plot stim", "update window", w453) -> (w439:string[])
          n182 = local write "wftab"(w437) -> ()
        }
        frame "update window" {
          n183 = Unbundle By Name(w464) -> ("Window.Type"=w463:T6)
          n184 = Not Equal?(x=w463, y=HRTF-Window_Type."None") -> (x != y?=w461:bool)
          n185 = property on="Length (ms)" class="DigNum (strict)"("Visible"=w461) -> ()  [unwired: 2 in, 2 out]
          n186 = property on="Center (ms)" class="DigNum (strict)"("Visible"=w461) -> ()  [unwired: 2 in, 2 out]
        }
        frame "plot stim" {
          n187 = call "SAC-Create Stimulus.vi"("Params"=w474) -> ("duration (ms)"=→"StimDur":dbl, "time"=→"Stimulus (time)":cluster{i32, "dx":dbl, "Y":dbl[]}, "autocorr"=→"StimAutocorr":cluster{dbl, "dx":dbl, "Y":dbl[]}, "mag"=→"StimMag":cluster{i32, "dx":dbl, "Y":dbl[]}, "phase"=→"StimPhase":cluster{i32, "dx":dbl, "Y":dbl[]})  [unwired: 9 in, 1 out]
          n188 = local write "Data Tab"(enum32{"Stimulus", "Response", "Calibrations"}."Stimulus" ("Data Tab")) -> ()
        }
        frame "do next" {
          n189 = invoke on="Config" class="SAC Config (strict)" method="Select next.vi"() -> ("Select next.vi"=w479:i32)  [unwired: 3 in, 2 out]
          n190 = Unbundle By Name(w481) -> ("Azimuths"=w480:dbl[])
          n191 = Index Array(array=w480, index=w479) -> (element=w478:dbl)
          n192 = Bundle By Name(cluster=w485, "Azimuth"=w478, "iAzimuth"=w479) -> (w484:T8)
          n193 = case shown="0, Default" w479 {
            tunnel: w487 -> [w494 _]
            tunnel: w481 -> [w493 _]
            tunnel: w486 -> [w492 _]
            tunnel: w484 -> [w490 _]
            tunnel: [_ string[] ["end run"] ("String")] -> w483
            tunnel: [w488 u8 0] -> w482
            frame 0, Default {
              n194 = property on="Progress" class="Slide (strict)"() -> ("Value"=w489:u8)  [unwired: 2 in, 2 out]
              n195 = Bundle("Options"=w493, "Params"=w492, "State"=w490) -> (w491:cluster{"Options":T7, "Params":T3, "State":T8})  [unwired: 1 in]
              n196 = Increment(x=w489) -> (x+1=w488:u8)
              n197 = Enqueue Element(queue=w494, element=w491) -> ()  [unwired: 2 in, 3 out]
            }
            frame -1 {
            }
          }
          n198 = property on="Progress" class="Slide (strict)"("Value"=w482) -> ()  [unwired: 2 in, 2 out]
        }
        frame "update" {
          n199 = Unbundle By Name(w499) -> ("Azimuths"=w498:dbl[])
          n200 = Unbundle By Name(w500) -> ("iAzimuth"=w501:i32)
          n201 = property on="Config" class="SAC Config (strict)"("completed"=w501) -> ()  [unwired: 2 in, 2 out]
          n202 = call "SAC-Enum Data Files.vi"("Azimuths"=w498) -> ("file status"=w497:bool[])  [unwired: 13 in, 1 out]
          n203 = disable-structure shown="Disabled" {
            disable-tunnel: w497 -> [w504 _]
            frame Disabled {
              n204 = property on="Config" class="SAC Config (strict)"("file status"=w504) -> ()  [unwired: 2 in, 2 out]
            }
            frame Enabled {
            }
          }
        }
        frame "enum work" {
          n205 = Unbundle By Name(w512) -> ("Azimuths"=w511:dbl[])
          n206 = call "SAC-Enum Data Files.vi"("State"=w505, "Azimuths"=w511) -> ("filestems"=w510:string[], "file status"=w506:bool[])  [unwired: 12 in]
          n207 = Build Array (concatenate)("", w510) -> (w508:string[])
          n208 = property on="Config" class="SAC Config (strict)"("file status"=w506) -> ()  [unwired: 2 in, 2 out]
          n209 = property on="RespFiles" class="Ring (strict)"("Strings []"=w508, "Value"=0) -> ()  [unwired: 2 in, 2 out]
        }
        frame "enum astfs" {
          n210 = Unbundle By Name(w522) -> ("Azimuths"=w521:dbl[])
          n211 = call "SAC-Enum Data Files.vi"("State"=w515, "Azimuths"=w521, "ASTFs"=TRUE ("HRTFs")) -> ("filestems"=w520:string[])  [unwired: 11 in, 1 out]
          n212 = Build Array (concatenate)("", w520) -> (w517:string[])
          n213 = property on="ASTFFiles" class="Ring (strict)"("Strings []"=w517, "Value"=0) -> ()  [unwired: 2 in, 2 out]
        }
        frame "read work" {
          n214 = local read "RespFiles"() -> (w531:u16)
          n215 = property on="RespFiles" class="Ring (strict)"() -> ("Strings []"=w532:string[])  [unwired: 2 in, 2 out]
          n216 = Index Array(array=w532, index=w531) -> (element=w530:string)
          n217 = case shown="\"True\", Default" w530 {
            selector: w530 -> [_ w541]
            tunnel: w529 -> [_ w536]
            tunnel: [_ w540] -> w528
            tunnel: [_ w539] -> w527
            tunnel: [_ w538] -> w526
            tunnel: [_ w537] -> w525
            frame "" {
            }
            frame "True", Default {
              n218 = call "SAC-Read Responses.vi"("State"=w536, "filestem"=w541) -> ("time"=w540:cluster{"offset":dbl, "dx":dbl, "Y":dbl[]}, "crosscorr"=w539:cluster{"offset":dbl, "dx":dbl, "Y":dbl[]}, "phase"=w537:cluster{"offset":dbl, "dx":dbl, "Y":dbl[]}, "mag"=w538:cluster{"offset":dbl, "dx":dbl, "Y":dbl[]})  [unwired: 9 in, 1 out]
            }
          }
          n219 = local write "RespCorr"(w527) -> ()
          n220 = local write "RespMag"(w526) -> ()
          n221 = local write "RespPhase"(w525) -> ()
          n222 = local write "RespTime"(w528) -> ()
        }
        frame "read astf" {
          n223 = property on="ASTFFiles" class="Ring (strict)"() -> ("RingText.Text"=w544:string)  [unwired: 2 in, 2 out]
          n224 = case shown="\"True\", Default" w544 {
            selector: w544 -> [_ w554]
            tunnel: w546 -> [_ w550]
            tunnel: [_ w553] -> w545
            tunnel: [_ w552] -> w543
            tunnel: [_ w551] -> w542
            frame "" {
            }
            frame "True", Default {
              n225 = call "SAC-Read ASTFs.vi"("State"=w550, "filestem"=w554) -> ("IR"=w553:cluster{"offset":dbl, "dx":dbl, "Y":dbl[]}, "phase"=w551:cluster{dbl, "dx":dbl, "Y":dbl[]}, "mag"=w552:cluster{dbl, "dx":dbl, "Y":dbl[]})  [unwired: 10 in, 1 out]
            }
          }
          "ASIR" <- w545
          "ASTFMag" <- w543
          "ASTFPhase" <- w542
        }
        frame "show astf" {
          n226 = call "SAC-Build Matfile Path.vi"("State"=w566) -> ("filestem"=w565:string)  [unwired: 13 in, 1 out]
          n227 = property on="ASTFFiles" class="Ring (strict)"() -> ("Strings []"=w560:string[])  [unwired: 2 in, 2 out]
          n228 = Array Size(array=w560) -> (size(s)=w559:i32)
          n229 = Search 1D Array(1D array=w560, element=w565) -> (index of element=w564:i32)  [unwired: 1 in]
          n230 = Greater?(x=w559, y=1) -> (0:w557:bool)
          n231 = Boolean To (0,1)(Boolean=w557) -> (0, 1=w556:i16)
          n232 = Max & Min(x=w564, y=w556) -> (max(x,y)=w563:i32)  [unwired: 1 out]
          n233 = local write "Data Tab"(enum32{"Stimulus", "Response", "Calibrations"}."Calibrations" ("Data Tab")) -> ()
          n234 = property on="ASTFFiles" class="Ring (strict)"("Value"=w563) -> ()  [unwired: 2 in, 2 out]
          n235 = Build Array (concatenate)(w567, "read astf") -> (w562:string[])
        }
        frame "end run" {
          n236 = property on="Config" class="SAC Config (strict)"("highlight"=-1) -> ("selection"=w574:i32[])  [unwired: 2 in, 2 out]
          n237 = Array Size(array=w574) -> (size(s)=w573:i32)
          n238 = Greater Than 0?(x=w573) -> (x > 0?=w571:bool)
          n239 = call "Enable or Gray Out.vi"("Boolean"=w571) -> ("Disabled"=w570:T10)
          n240 = property on="Start" class="Bool"("Visible"=TRUE, "DisabledEnum"=w570) -> ()  [unwired: 2 in, 2 out]
          n241 = property on="RespFiles" class="Ring (strict)"("DisabledEnum"=T10."Enabled" ("Disabled")) -> ()  [unwired: 2 in, 2 out]
          n242 = property on="Status" class="Str"("Visible"=FALSE) -> ()  [unwired: 2 in, 2 out]
        }
        frame "enable start" {
          n243 = property on="Config" class="SAC Config (strict)"() -> ("selection"=w582:i32[])  [unwired: 2 in, 2 out]
          n244 = Unbundle By Name(w584) -> ("Folder"=w588:path)
          n245 = Array Size(array=w582) -> (size(s)=w585:i32)
          n246 = call "FileIO-File or Folder Exists.vi"("path"=w588) -> ("Exists?"=w589:bool)  [unwired: 7 in, 3 out]
          n247 = Greater Than 0?(x=w585) -> (x > 0?=w586:bool)
          n248 = Compound Arithmetic op=AND(w589, w586) -> (w587:bool)
          n249 = call "Enable or Gray Out.vi"("Boolean"=w587) -> ("Disabled"=w583:T10)
          n250 = property on="Start" class="Bool"("DisabledEnum"=w583) -> ()  [unwired: 2 in, 2 out]
        }
        frame "compute" {
          w594 = T10."Enabled" ("Disabled")
          n251 = Unbundle By Name(w601) -> ("Fs (Hz)"=w600:dbl)
          n252 = control-ref of="Progress"() -> (w599:refnum<vi>)
          n253 = call "SAC-Compute ASTFs.vi"("State"=w593, "Progress"=w599, "Window"="Window", "Desired Fs"=w600) -> ("error out"=w598:errorcluster)  [unwired: 11 in]
          n254 = call "Error Handler.vi"("error in (no error)"=w598) -> ("No Error"=w597:errorcluster)  [unwired: 13 in, 1 out]
          n255 = property on="Compute" class="Bool"(error in=w597, "DisabledEnum"=w594) -> ()  [unwired: 1 in, 2 out]
          n256 = property on="Start" class="Bool"("DisabledEnum"=w594) -> ()  [unwired: 2 in, 2 out]
          n257 = Build Array (concatenate)(w603, string[] ["show astf", "enum astfs"] ("array")) -> (w596:string[])
        }
      }
      n258 = Empty Array?(array=w387) -> (empty?=w386:bool)
    }
  }
  n259 = while {
    tunnel: w14 -> [w608]
    tunnel: w11 -> [w605]
    stop <- w607 stop-if-true
    # "MEASUREMENT THREAD"
    n260 = Dequeue Element(queue=w608) -> (element=w606:cluster{"Options":T7, "Params":T3, "State":T8}, error out=w607:errorcluster)  [unwired: 2 in, 2 out]
    n261 = case shown="No Error" w607 {
      tunnel: w606 -> [w617 _]
      tunnel: w605 -> [w613 _]
      frame No Error {
        n262 = Unbundle By Name(w617) -> ("Options"=w616:T7, "Params"=w615:T3, "State"=w614:T8)
        n263 = while {
          shift-right: [w630] -> _
          shift-left: w616 -> [w633]
          shift-right: [w629] -> _
          shift-left: w615 -> [w632]
          shift-right: [w628] -> _
          shift-left: w614 -> [w631]
          tunnel: w613 -> [w626]
          shift-right: [w624] -> _
          shift-left: errorcluster {"status"=FALSE, "code"=0, "source"=""} ("error constant") -> [w625]
          shift-right: [w623] -> _
          shift-left: T18 {"StimSpec"=[], "Mic Sum"=[], "df (Hz)"=0.0, "dt (ms)"=0.0, "Navg"=0, "Nacq"=0, "pts/rep"=0, "reps/frame"=0, "Stimulus"=[]} ("Cal.Data") -> [w622]
          shift-right: [w620] -> _
          shift-left: T2 {"error"={"status"=FALSE, "code"=0, "source"=""}, "aborted"=FALSE} ("Value (Signaling)") -> [w621]
          shift-right: [w618] -> _
          shift-left: HRTF-State_Machine_Action."Wait" ("Action") -> [w619]
          stop <- w627 stop-if-true
          n264 = case shown="\"Init\"" w619 {
            tunnel: w633 -> [w651 w677 w710 w736 w773 w783]
            tunnel: w632 -> [w652 w655 w709 w733 w763 w782]
            tunnel: w631 -> [w634 w661 w700 w725 w758 w781]
            tunnel: [w651 w677 w710 w736 w773 w783] -> w630
            tunnel: [w652 w655 w709 w733 w763 w782] -> w629
            tunnel: [w634 w661 w700 w725 w758 w781] -> w628
            tunnel: [_ _ _ _ _ TRUE] -> w627
            tunnel: w626 -> [w650 _ _ w731 _ _]
            tunnel: [w647 w672 w705 w728 HRTF-State_Machine_Action."End" ("Action") HRTF-State_Machine_Action."End" ("Action")] -> w618
            tunnel: w625 -> [w642 w675 w702 w735 w764 w777]
            tunnel: [w642 w674 w701 w726 w759 w777] -> w624
            tunnel: [w640 w662 w704 w721 w769 w776] -> w623
            tunnel: w622 -> [w640 _ w704 w732 w769 w776]
            tunnel: w621 -> [w639 w658 w703 w723 w770 w775]
            tunnel: [w638 w658 w703 w722 w770 w775] -> w620
            frame "Wait" {
              n265 = local write "Status"("Waiting..." ("Status")) -> ()
              n266 = Unbundle By Name(w651) -> ("Wait (s)"=w644:dbl)
              n267 = call "SAC-Build Filename.vi"("State"=w634) -> ("filestem"=w636:string)  [unwired: 13 in, 1 out]
              n268 = control-ref of="RespFiles"() -> (w637:refnum<vi>)
              n269 = call "X1000.vi"("X"=w644) -> ("X/1000"=w643:dbl)
              n270 = call "SAC-Add Filestem to Ring.vi"("Ring in"=w637, "filename"=w636) -> ()  [unwired: 14 in]
              n271 = local write "Data Tab"(enum32{"Stimulus", "Response", "Calibrations"}."Response" ("Data Tab")) -> ()
              n272 = Wait on Notification(notifier=w650, timeout in ms (-1)=w643) -> (timed out?=w645:bool)  [unwired: 2 in, 3 out]
              n273 = Not(x=w645) -> (.not. x?=w641:bool)
              n274 = Bundle By Name(cluster=w639, "aborted"=w641) -> (w638:T2)
              n275 = Select(t=HRTF-State_Machine_Action."End" ("Action"), s=w641, f=HRTF-State_Machine_Action."Init") -> (s? t:f=w647:T19)
            }
            frame "Init" {
              n276 = disable-structure shown="HARDWARE==TDT" {
                disable-tunnel: w675 -> [w684 w691]
                disable-tunnel: [w683 w685] -> w674
                disable-tunnel: [w682 w686] -> w669
                disable-tunnel: [w681 w688] -> w656
                disable-tunnel: w655 -> [w680 w690]
                disable-tunnel: [w679 w687] -> w654
                disable-tunnel: [w678 w689] -> w657
                frame condition #0 {
                  n277 = call "SAC-Configure Hardware (NI).vi"("Params"=w680, "error in (no error)"=w684) -> ("Stimulus"=w678:dbl[], "Sample Rate (Hz)"=w681:dbl, "pts/rep"=w679:i32, "reps/frame"=w682:i32, "error out"=w683:errorcluster)  [unwired: 9 in]
                }
                frame condition #1 (active) {
                  n278 = call "SAC-Configure Hardware (TDT).vi"("Params"=w690, "error in (no error)"=w691) -> ("Stimulus"=w689:dbl[], "Sample Rate (Hz)"=w688:dbl, "pts/rep"=w687:i32, "reps/frame"=w686:i32, "error out"=w685:errorcluster)  [unwired: 9 in]
                }
              }
              n279 = local write "Status"("Initializing..." ("Status")) -> ()
              n280 = Unbundle By Name(w655) -> ("Averages"=w660:i32)
              n281 = Reverse 1D Array(array=w657) -> (reversed array=w659:dbl[])
              n282 = call-poly <vilib>:"FFT.vi"("X"=w659) -> ("FFT {X}"=w653:cdb[])  [unwired: 9 in, 1 out]
              n283 = Initialize Array(0.0 ("element"), w654) -> (w663:dbl[])
              n284 = Divide(x=1000.0, y=w656) -> (x/y=w668:dbl)
              n285 = Divide(x=w656, y=w654) -> (x/y=w666:dbl)
              n286 = Bundle By Name(cluster=T18 {"StimSpec"=[], "Mic Sum"=[], "df (Hz)"=0.0, "dt (ms)"=0.0, "Navg"=0, "Nacq"=0, "pts/rep"=0, "reps/frame"=0, "Stimulus"=[]} ("Cal.Data"), "StimSpec"=w653, "Stimulus"=w657, "pts/rep"=w654, "reps/frame"=w669, "dt (ms)"=w668, "df (Hz)"=w666, "Nacq"=0, "Mic Sum"=w663, "Navg"=w660) -> (w662:T18)
              n287 = Select(t=HRTF-State_Machine_Action."End" ("Action"), s=w674, f=HRTF-State_Machine_Action."Multiplex") -> (s? t:f=w672:T19)
            }
            frame "Multiplex" {
              w695 = T16 {"Output"={"Device"=enum."None", "Num"=0}, "Speaker"={"Channel"=0, "Primary mux"=0, "Secondary mux"=1}, "Cal mic"=0} ("TDT")
              n288 = call "Config File Path.vi"() -> ("Default config file name"=w696:path)  [unwired: 1 in]
              n289 = local write "Status"("Multiplexing..." ("Status")) -> ()
              n290 = Unbundle By Name(w700) -> ("iAzimuth"=w699:i32)
              n291 = call "Read Anything.vi"("Type of Anything"=w695, "Section Name (Name of \"Type of Anything\")"="TDT Config" ("Section Name (Name of \"Type of Anything\")"), "Path (dialog)"=w696) -> ("Anything"=w698:variant)  [unwired: 6 in, 2 out]
              n292 = Variant To Data(type=w695, Variant=w698) -> (data=w694:T16)  [unwired: 1 in, 1 out]
              n293 = Unbundle By Name(w694) -> ("Speaker.Primary mux"=w693:i32, "Speaker.Secondary mux"=w692:i32)
              n294 = disable-structure shown="HARDWARE==TDT" {
                disable-tunnel: w702 -> [w711 w714]
                disable-tunnel: [w711 w718] -> w701
                disable-tunnel: w699 -> [_ w717]
                disable-tunnel: w693 -> [_ w716]
                disable-tunnel: w692 -> [_ w715]
                frame condition #0 {
                  n295 = Wait (ms)(milliseconds to wait=u32 1000) -> ()  [unwired: 1 out]
                }
                frame condition #1 (active) {
                  n296 = call "TDT-Run Circuit.vi"("error in (no error)"=w714) -> ("error out"=w713:errorcluster)  [unwired: 14 in]
                  n297 = call "HRTF-Set Multiplexer (TDT).vi"("iAzimuth"=w717, "MUX 1"=w716, "MUX 2"=w715, "error in (no error)"=w713) -> ("error out"=w718:errorcluster)  [unwired: 11 in]
                }
              }
              n298 = Select(t=HRTF-State_Machine_Action."End" ("Action"), s=w701, f=HRTF-State_Machine_Action."Measure") -> (s? t:f=w705:T19)
            }
            frame "Measure" {
              n299 = call "SGDA-Start.vi"("error in (no error)"=w735) -> ("error out"=w734:errorcluster)  [unwired: 6 in]
              n300 = while {
                shift-right: [w742] -> w721
                shift-left: w732 -> [w756]
                shift-right: [w741] -> w726
                shift-left: w734 -> [w757]
                tunnel: w731 -> [w751]
                tunnel: [w748] -> w724
                i -> [w747]
                stop <- w749 stop-if-true
                n301 = call "SGDA-Read Data.vi"("error in (no error)"=w757) -> ("AI Waveforms"=w745:dbl[][], "error out"=w755:errorcluster)  [unwired: 13 in]
                n302 = Wait on Notification(notifier=w751, timeout in ms (-1)=0) -> (timed out?=w752:bool)  [unwired: 2 in, 3 out]
                n303 = Equal To 0?(x=w747) -> (x = 0?=w746:bool)
                n304 = Not(x=w752) -> (.not. x?=w748:bool)
                n305 = call "SAC-Process Frame.vi"("Cal.Data In"=w756, "AI Waveforms"=w745, "First"=w746, "error in (no error)"=w755) -> ("Cal.Data Out"=w743:T18, "Status"=w754:string, "Finished"=w753:bool, "error out"=w744:errorcluster)  [unwired: 8 in]
                n306 = local write "Status"(w754) -> ()
                n307 = call "SAC-Plot Response.vi"("Cal.Data in"=w743, "error in (no error)"=w744) -> ("Cal.Data out"=w742:T18, "time"=→"RespTime":cluster{"offset":dbl, "dx":dbl, "Y":dbl[]}, "crosscorr"=→"RespCorr":cluster{"offset":dbl, "dx":dbl, "Y":dbl[]}, "phase"=→"RespPhase":cluster{"offset":dbl, "dx":dbl, "Y":dbl[]}, "mag"=→"RespMag":cluster{"offset":dbl, "dx":dbl, "Y":dbl[]}, "error out"=w741:errorcluster)  [unwired: 8 in]
                n308 = Compound Arithmetic op=OR(w741, w753, w748) -> (w749:bool)
              }
              n309 = call "SGDA-Stop.vi"("error in (no error)"=w726) -> ("error out"=w720:errorcluster)  [unwired: 14 in]
              n310 = Or(x=w726, y=w724) -> (x .or. y?=w727:bool)
              n311 = call "TDT-Close ActiveX.vi"("error in (no error)"=w720) -> ("error out"=w719:errorcluster)  [unwired: 14 in]
              n312 = Bundle By Name(cluster=w723, "aborted"=w724) -> (w722:T2)
              n313 = call <vilib>:"Clear Errors.vi"("error in (no error)"=w719) -> ()  [unwired: 5 in, 2 out]
              n314 = Select(t=HRTF-State_Machine_Action."End" ("Action"), s=w727, f=HRTF-State_Machine_Action."Save") -> (s? t:f=w728:T19)
            }
            frame "Save" {
              n315 = Unbundle By Name(w769) -> ("Mic Sum"=w768:dbl[], "Nacq"=w767:i32, "Stimulus"=w765:dbl[], "dt (ms)"=w762:dbl)
              n316 = local write "Status"("Saving..." ("Status")) -> ()
              n317 = Divide(x=w768, y=w767) -> (x/y=w766:dbl[])
              n318 = call "Divide By 1000.vi"("X"=w762) -> ("X/1000"=w761:dbl)
              n319 = Reciprocal(x=w761) -> (1/x=w760:dbl)
              n320 = call "SAC-Write Text File.vi"("Params"=w763, "State"=w758, "Data"=w766, "Stimulus"=w765, "error in (no error)"=w764, "Actual Fs"=w760) -> ("error out"=w759:errorcluster)  [unwired: 9 in]
            }
            frame "End", Default {
              n321 = local write "Status"("Done." ("Status")) -> ()
              n322 = Bundle By Name(cluster=w775, "error"=w777) -> (w778:T2)
              n323 = property on="Result" class="Clust (strict)"("Val(Sgnl)"=w778) -> ()  [unwired: 2 in, 2 out]
            }
          }
        }
      }
      frame Error {
      }
    }
  }
